vi "Config Panel.vi"(7 "Error In":errorcluster, 10 "MSX-E3711 in":refnum<class "MSX-E3711.lvclass">=refnum) -> (0 "Error Out":errorcluster, 3 "MSX-E3711 out":refnum<class "MSX-E3711.lvclass">)   [LabVIEW 2014, in "MSX-E3711.lvlib" / "MSX-E3711.lvclass"]
doc: "PANEL FRONTAL PARA PRICIPAL DE CONFIGURACION."
uses:
  MSX-E3711Class/MSX-E3711.lvclass
  MSX-E3711Class/MSX-E3711.lvclass/MSX-E3711.ctl
  DriverMasterSync/build/DriverMasterSync.lvlibp/Modules/HAL/DriverMasterSync/DriverMasterSyncClass/DriverMasterSync.lvclass
  API/MSX-E3711_dll.lvlib
panel:
  in  "TempConf":bool
  in  "CountConf":bool
  in  "Activar Temp":bool
  in  "Activar Count":bool
  in  "Activar  Count":bool
  in  "Activar  Temp":bool
  in  "Aplicar":bool
  in  "Cancelar":bool
  in  "Aceptar":bool
  in  "Protection":bool
  in  "Transducer Selection":bool
  in  "Offset":bool
  in  "Gain":bool
  in  "Diagnostic":bool
  in  "Calibration":bool
  in  "Transductores":bool[][](array[boolean])=[[TRUE, FALSE, FALSE, FALSE], [FALSE, FALSE, FALSE, FALSE], [FALSE, FALSE, FALSE, FALSE], [FALSE, FALSE, FALSE, FALSE]]
  in  "Nbr Of Sequence":u64
  in  "Nbr Max Seq To Transfer":u64=800
  in  "Connection Data.IP":string="192.168.2.98"
  # "ADDI-DATA MSX-E3711"
  # "IP Config"
  # "Sequence"
  # "AutoRefresh"
  # "1"
  # "2"
  # "3"
  # "4"
  # "5"
  # "6"
  # "7"
  # "8"
  # "Configuración"
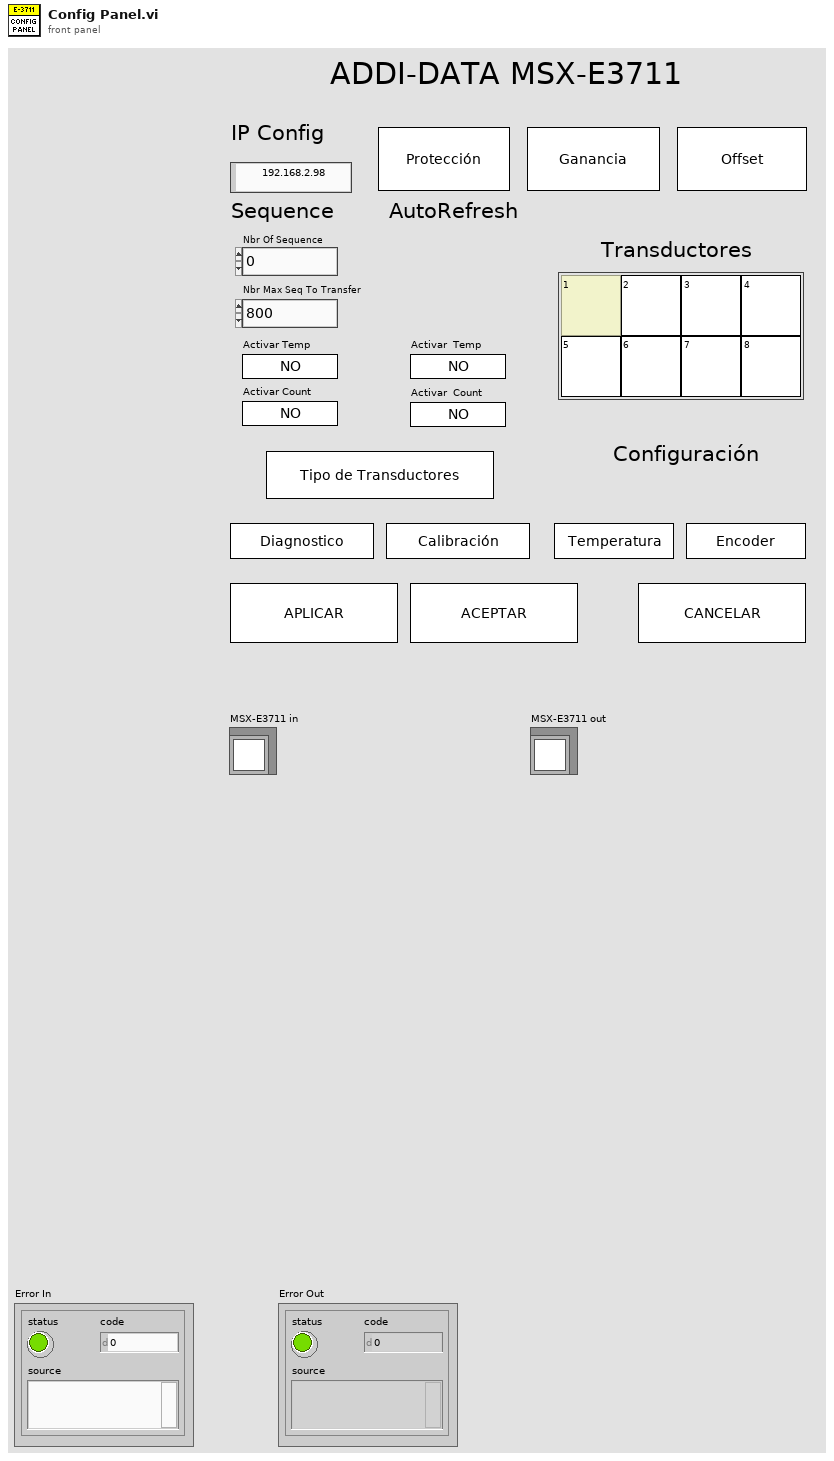
[diagram p1: front panel]
types:
  T1 = typedef "DriverMasterSync.lvlibp/HAL Config Data.ctl" = cluster{"HWSync Index":u32, "Driver Name":string, "Channel Mask":u64}
  T2 = typedef "MSX-E3711_dll.lvlib/Config Data.ctl" = cluster{"Auto Refresh":cluster{"Average Mode":u64, "Average Value":u64, "Trigger Mask":u64, "Trigger Mode":u64, "Hardware Trigger Edge":u64, "Hardware Trigger Count":u64, "By Trigger Nbr Of Seq To Acquire":u64, "Time stamp":bool, "Analog Output(mm)":bool, "Invert value":bool, "Temperature value":bool, "Incremental counter value":bool, "Diff. mode":bool}, "Gain":sgl[], "Offset":sgl[], "Index":u64, "Range":sgl, "Sequence":cluster{"Nbr Of Sequence":u64, "Nbr Max Sequence To Transfer":u64, "Delay Mode":u64, "Delay Time Unit":u64, "Delay Value":u64, "Trigger Mask":u64, "Trigger Mode":u64, "Hardware Trigger Edge":u64, "Hardware Trigger Count":u64, "By Trigger Nbr Of Seq To Acquire":u64, "Time stamp":bool, "Sequence counter information":bool, "Analog Output(mm)":bool, "Invert value":bool, "Temperature value":bool, "Incremental counter value":bool, "Diff. mode":bool}, "Enable DIO":bool, "IncCounter":cluster{"CounterMode":string, "CounterOptionDIRECT  ":bool, "CounterOptionOthers":bool, "CounterClear ":bool, "Cantidad de Pulsos":sgl, "Reducción":sgl}, "IncTemperature":cluster{"ConnectedTempSensor":string, "ConvertMode":string, "InitGainSelection":string, "FrequencySelection":string, "PowerSaveMode":bool, "GainSelection":string, "RefValue":dbl}}
  T3 = cluster{"Average Mode":u64, "Average Value":u64, "Trigger Mask":u64, "Trigger Mode":u64, "Hardware Trigger Edge":u64, "Hardware Trigger Count":u64, "By Trigger Nbr Of Seq To Acquire":u64, "Time stamp":bool, "Analog Output(mm)":bool, "Invert value":bool, "Temperature value":bool, "Incremental counter value":bool, "Diff. mode":bool}
  T4 = cluster{"Nbr Of Sequence":u64, "Nbr Max Sequence To Transfer":u64, "Delay Mode":u64, "Delay Time Unit":u64, "Delay Value":u64, "Trigger Mask":u64, "Trigger Mode":u64, "Hardware Trigger Edge":u64, "Hardware Trigger Count":u64, "By Trigger Nbr Of Seq To Acquire":u64, "Time stamp":bool, "Sequence counter information":bool, "Analog Output(mm)":bool, "Invert value":bool, "Temperature value":bool, "Incremental counter value":bool, "Diff. mode":bool}
  T5 = typedef "MSX-E3711_dll.lvlib/Connection Data.ctl" = cluster{"MX371x refnum":refnum<k24>, "IP":string, "Connection ID ":refnum<k5>, "MXCommon refnum":refnum<k24>}
  T6 = typedef "MSX-E3711_dll.lvlib/Diagnostic Data.ctl" = cluster{"Muestras Diag. Cycle":u32, "Tolerancia Cycle":sgl, "Tolerancia":sgl, "Mask Proteccion T":u64, "Promedio Transd":sgl[]}
  T7 = cluster{"ConnectedTempSensor":string, "ConvertMode":string, "InitGainSelection":string, "FrequencySelection":string, "PowerSaveMode":bool, "GainSelection":string, "RefValue":dbl}
  T8 = cluster{"CounterMode":string, "CounterOptionDIRECT  ":bool, "CounterOptionOthers":bool, "CounterClear ":bool, "Cantidad de Pulsos":sgl, "Reducción":sgl}
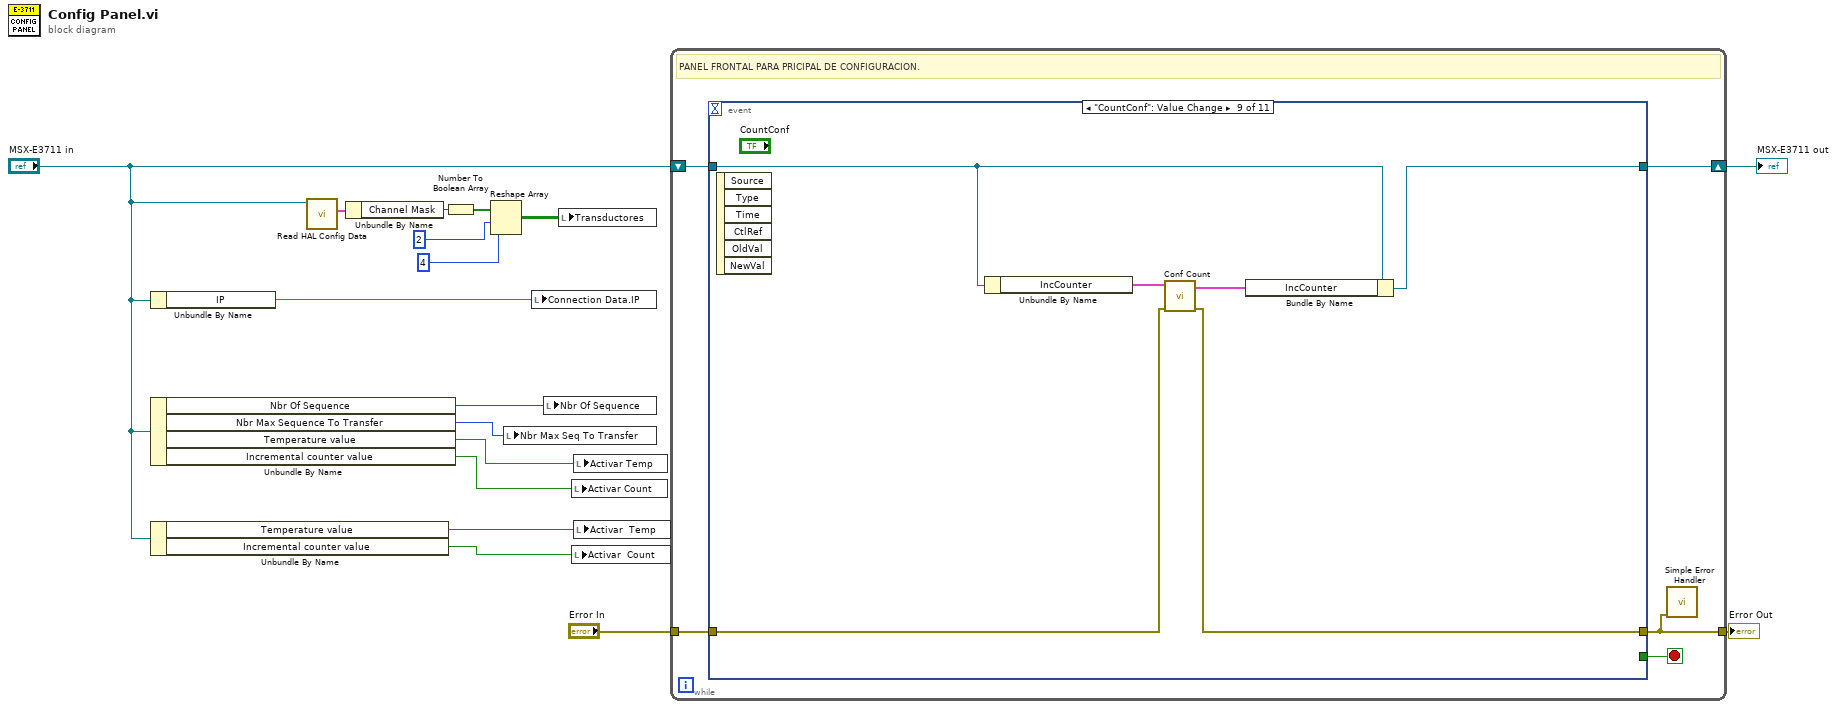
[diagram p0: block diagram]
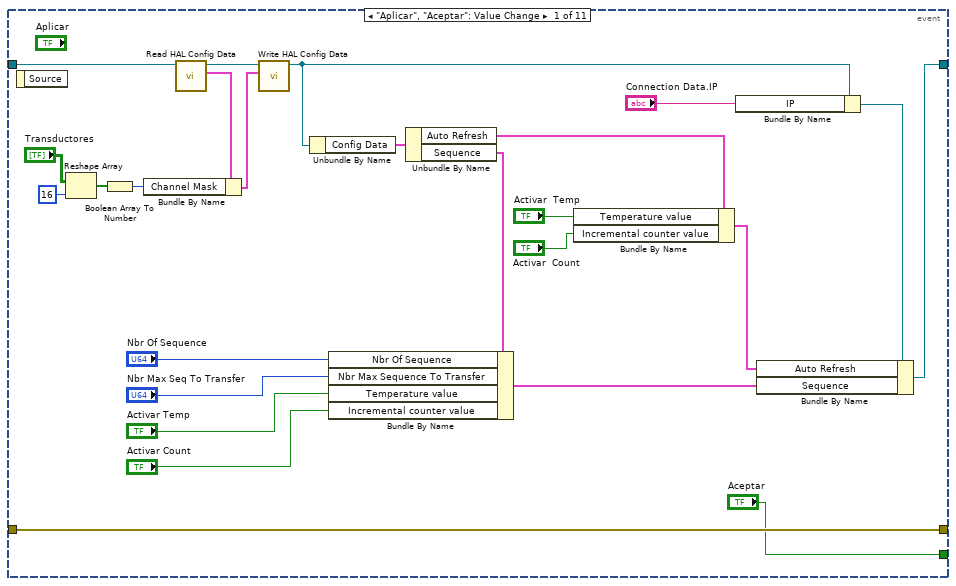
[diagram p2: hidden frame]
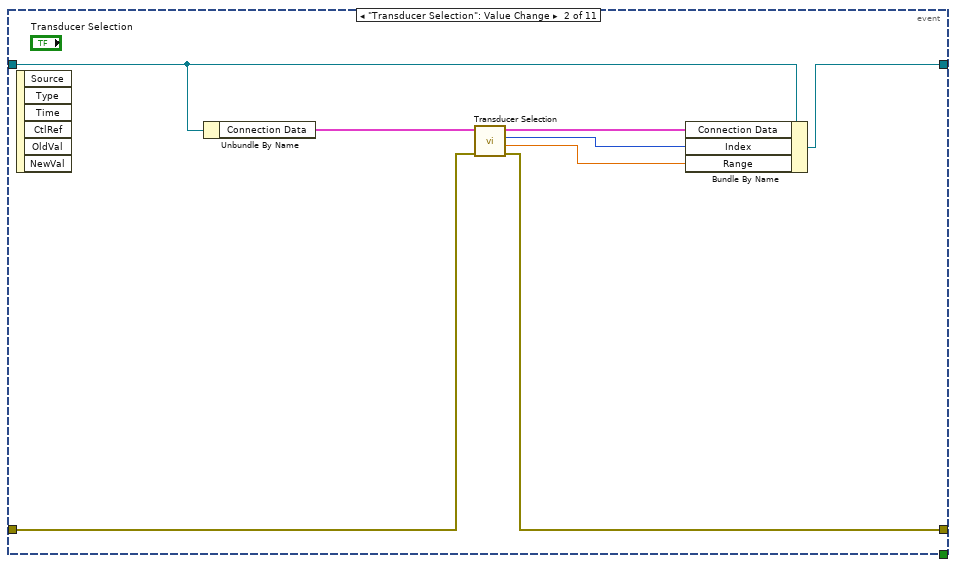
[diagram p3: hidden frame]
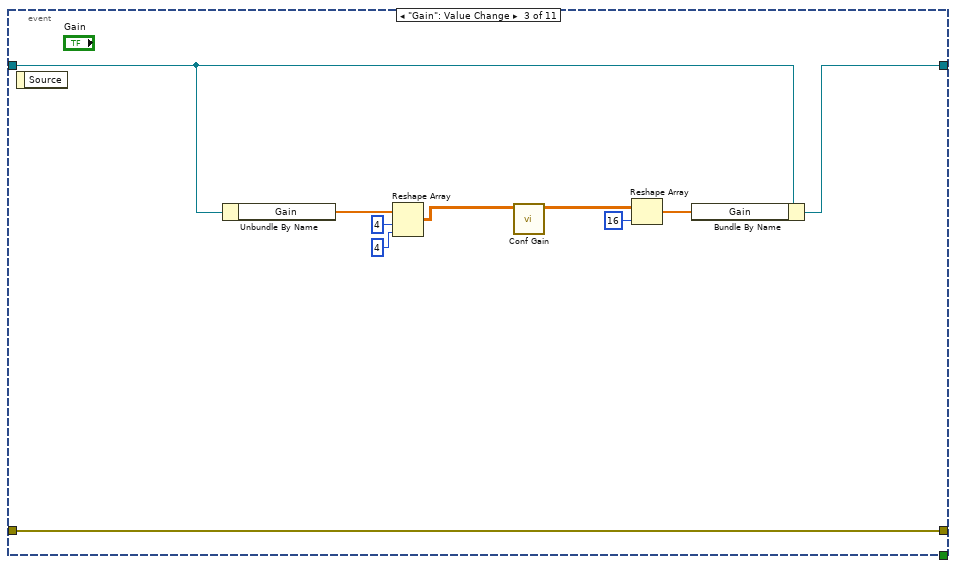
[diagram p4: hidden frame]
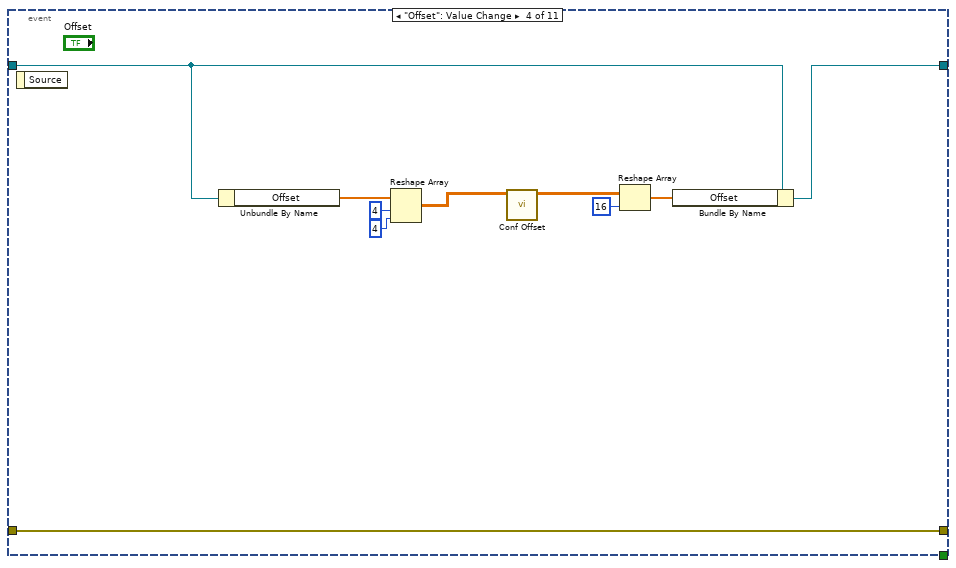
[diagram p5: hidden frame]
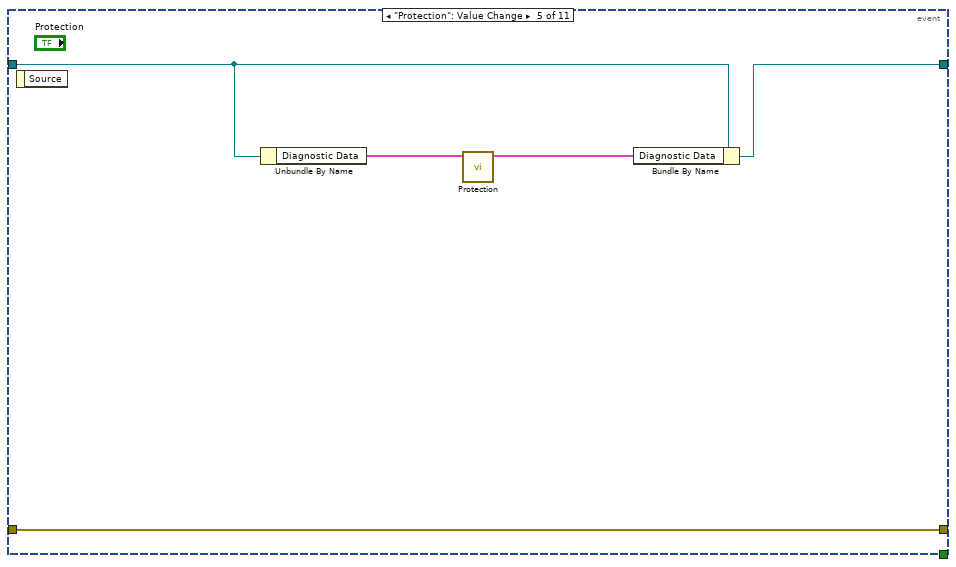
[diagram p6: hidden frame]
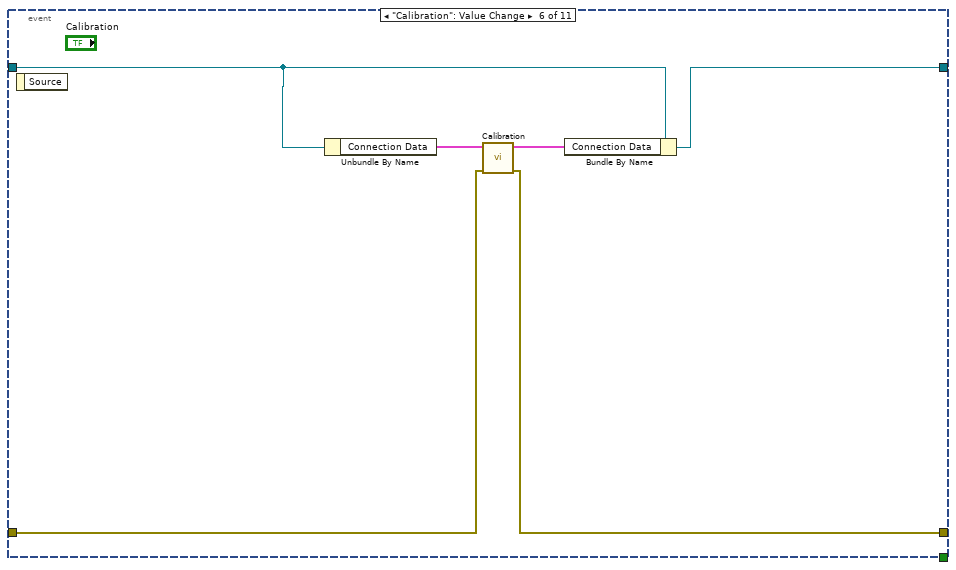
[diagram p7: hidden frame]
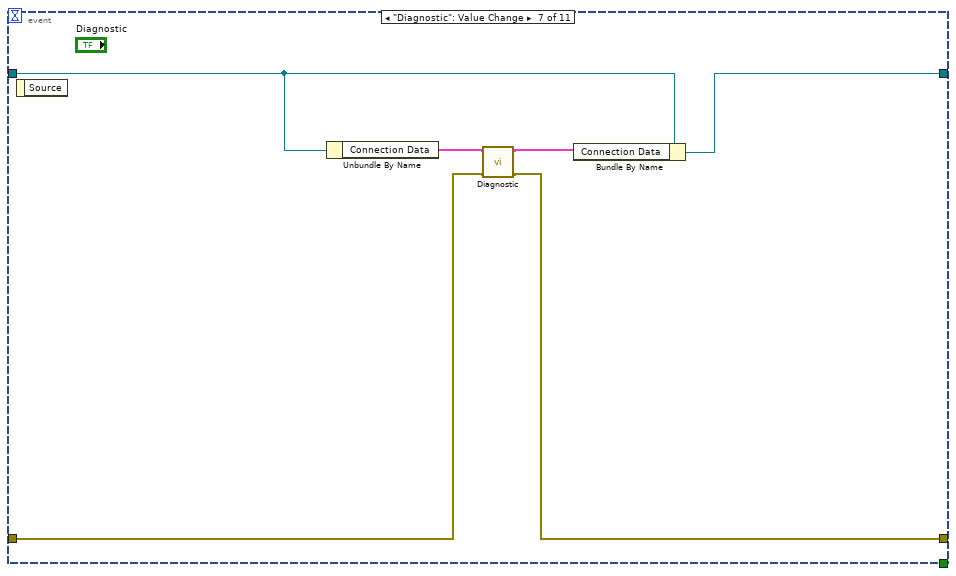
[diagram p8: hidden frame]
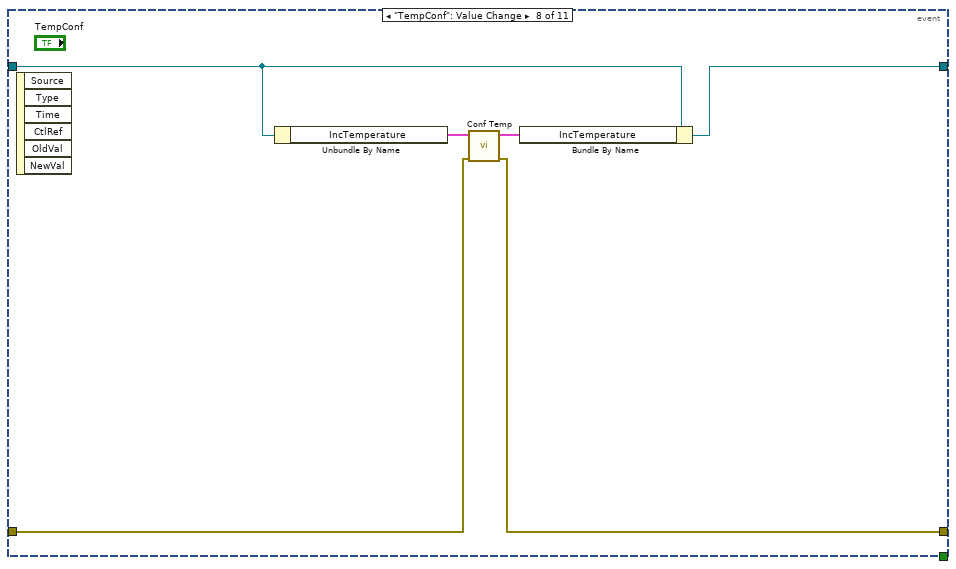
[diagram p9: hidden frame]
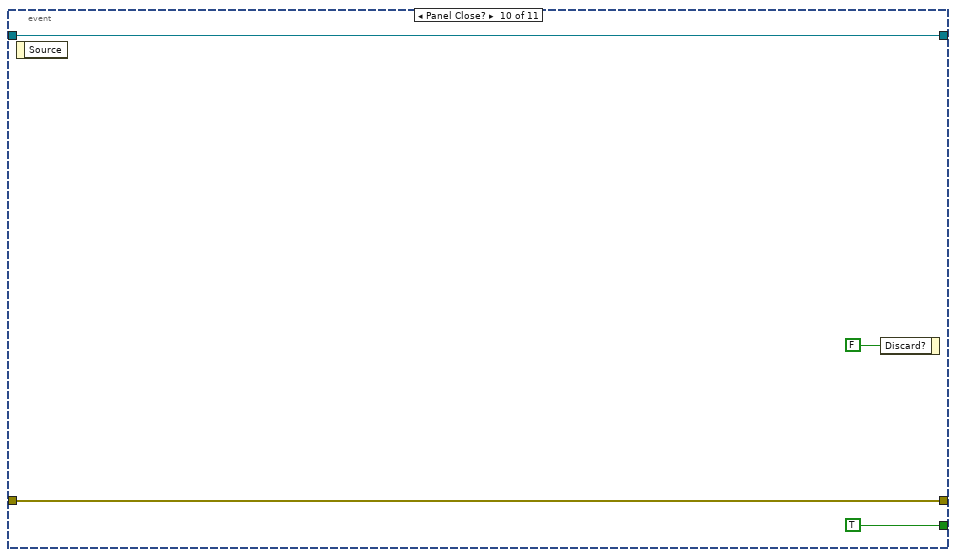
[diagram p10: hidden frame]
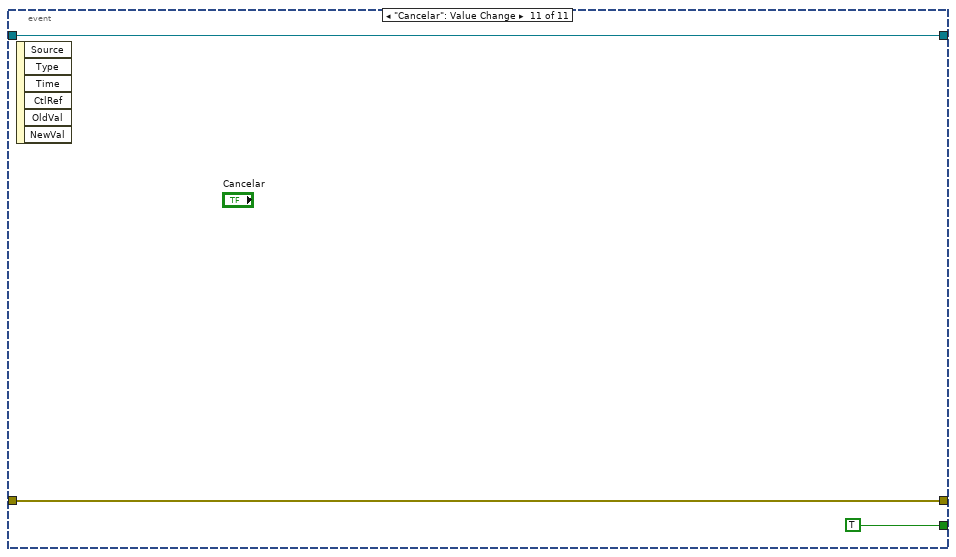
[diagram p11: hidden frame]
diagram:
  n1 = Unbundle By Name("MSX-E3711 in") -> ("IP"=w7:string)
  n2 = Unbundle By Name("MSX-E3711 in") -> ("Nbr Of Sequence"=w9:u64, "Nbr Max Sequence To Transfer"=w8:u64, "Temperature value"=w4:bool, "Incremental counter value"=w3:bool)
  n3 = Unbundle By Name("MSX-E3711 in") -> ("Temperature value"=w2:bool, "Incremental counter value"=w1:bool)
  n4 = call "Read HAL Config Data.vi"("DriverMasterSync in"="MSX-E3711 in") -> ("HAL Config Data"=w15:T1)  [unwired: 8 in, 2 out]
  n5 = Unbundle By Name(w15) -> ("Channel Mask"=w14:u64)
  n6 = Number To Boolean Array(number=w14) -> (Boolean array=w13:bool[])
  n7 = Reshape Array(w13, 2 ("dimension size"), 4 ("dimension size")) -> (w12:bool[][])
  n8 = local write "Nbr Max Seq To Transfer"(w8) -> ()
  n9 = local write "Connection Data.IP"(w7) -> ()
  n10 = local write "Nbr Of Sequence"(w9) -> ()
  n11 = local write "Transductores"(w12) -> ()
  n12 = local write "Activar Count"(w3) -> ()
  n13 = local write "Activar  Count"(w1) -> ()
  n14 = local write "Activar Temp"(w4) -> ()
  n15 = local write "Activar  Temp"(w2) -> ()
  n16 = while {
    tunnel: [w19] -> w17
    tunnel: "Error In" -> [w20]
    shift-right: [w18] -> w6
    shift-left: "MSX-E3711 in" -> [w21]
    stop <- w22 stop-if-true
    # "PANEL FRONTAL PARA PRICIPAL DE CONFIGURACION."
    n17 = event shown="[8] \"CountConf\": Value Change" {
      selector: _ -> [_ _ _ _ _ _ _ _ _ _ _]
      dyn-events: _ -> [_ _ _ _ _ _ _ _ _ _ _]
      timeout: _ -> [_ _ _ _ _ _ _ _ _ _ _]
      tunnel: ["Aceptar" _ _ _ _ _ _ _ _ TRUE ("Cancel Program") TRUE ("Cancel Program")] -> w22
      tunnel: [w45 w54 w63 w73 w78 w86 w91 w96 w99 w108 w111] -> w18
      tunnel: w21 -> [w33 w55 w64 w74 w79 w85 w92 w95 w100 w108 w111]
      tunnel: w20 -> [w39 w52 w65 w75 w80 w81 w87 w94 w103 w107 w110]
      tunnel: [w39 w51 w65 w75 w80 w82 w88 w93 w102 w107 w110] -> w19
      event "Aplicar", "Aceptar": Value Change {
        n18 = event-data() -> ()  [unwired: 1 in, 1 out]
        n19 = Reshape Array("Transductores", 16 ("dimension size")) -> (w38:bool[])
        n20 = Boolean Array To Number(Boolean array=w38) -> (number=w36:u64)
        n21 = call "Read HAL Config Data.vi"("DriverMasterSync in"=w33) -> ("HAL Config Data"=w30:T1, "DriverMasterSync out"=w32:refnum<class "MSX-E3711.lvclass">)  [unwired: 8 in, 1 out]
        n22 = Bundle By Name(cluster=w30, "Channel Mask"=w36) -> (w31:T1)
        n23 = call "Write HAL Config Data.vi"("HAL Config Data"=w31, "DriverMasterSync in"=w32) -> ("DriverMasterSync out"=w29:refnum<class "MSX-E3711.lvclass">)  [unwired: 8 in, 1 out]
        n24 = Unbundle By Name(w29) -> ("Config Data"=w46:T2)
        n25 = Unbundle By Name(w46) -> ("Auto Refresh"=w26:T3, "Sequence"=w41:T4)
        n26 = Bundle By Name(cluster=w41, "Nbr Of Sequence"="Nbr Of Sequence", "Nbr Max Sequence To Transfer"="Nbr Max Seq To Transfer", "Temperature value"="Activar Temp", "Incremental counter value"="Activar Count") -> (w40:T4)
        n27 = Bundle By Name(cluster=w26, "Temperature value"="Activar  Temp", "Incremental counter value"="Activar  Count") -> (w25:T3)
        n28 = Bundle By Name(cluster=w29, "IP"="Connection Data.IP") -> (w44:refnum<class "MSX-E3711.lvclass">)
        n29 = Bundle By Name(cluster=w44, "Auto Refresh"=w25, "Sequence"=w40) -> (w45:refnum<class "MSX-E3711.lvclass">)
      }
      event "Transducer Selection": Value Change {
        n30 = event-data() -> ()  [unwired: 1 in, 6 out]
        n31 = Unbundle By Name(w55) -> ("Connection Data"=w53:T5)
        n32 = call "Transducer Selection.vi"("error in (no error)"=w52, "Connection Data In"=w53) -> ("error out"=w51:errorcluster, "Range"=w48:dbl, "Index"=w49:u64, "Connection Data Out"=w50:T5)  [unwired: 5 in]
        n33 = Bundle By Name(cluster=w55, "Connection Data"=w50, "Index"=w49, "Range"=w48) -> (w54:refnum<class "MSX-E3711.lvclass">)
      }
      event "Gain": Value Change {
        n34 = event-data() -> ()  [unwired: 1 in, 1 out]
        n35 = Unbundle By Name(w64) -> ("Gain"=w62:sgl[])
        n36 = Reshape Array(w62, 4 ("dimension size"), 4 ("dimension size")) -> (w57:sgl[][])
        n37 = call "Conf Gain.vi"("Gain in"=w57) -> ("Gain Out"=w56:sgl[][])  [unwired: 10 in]
        n38 = Reshape Array(w56, 16 ("dimension size")) -> (w58:sgl[])
        n39 = Bundle By Name(cluster=w64, "Gain"=w58) -> (w63:refnum<class "MSX-E3711.lvclass">)
      }
      event "Offset": Value Change {
        n40 = event-data() -> ()  [unwired: 1 in, 1 out]
        n41 = Unbundle By Name(w74) -> ("Offset"=w69:sgl[])
        n42 = Reshape Array(w69, 4 ("dimension size"), 4 ("dimension size")) -> (w67:sgl[][])
        n43 = call "Conf Offset.vi"("Offset in"=w67) -> ("Offset Out"=w66:sgl[][])  [unwired: 10 in]
        n44 = Reshape Array(w66, 16 ("dimension size")) -> (w68:sgl[])
        n45 = Bundle By Name(cluster=w74, "Offset"=w68) -> (w73:refnum<class "MSX-E3711.lvclass">)
      }
      event "Protection": Value Change {
        n46 = event-data() -> ()  [unwired: 1 in, 1 out]
        n47 = Unbundle By Name(w79) -> ("Diagnostic Data"=w77:T6)
        n48 = call "Protection.vi"("Diagnostic Data"=w77) -> ("Diagnostic Data out"=w76:T6)  [unwired: 10 in]
        n49 = Bundle By Name(cluster=w79, "Diagnostic Data"=w76) -> (w78:refnum<class "MSX-E3711.lvclass">)
      }
      event "Calibration": Value Change {
        n50 = event-data() -> ()  [unwired: 1 in, 1 out]
        n51 = Unbundle By Name(w85) -> ("Connection Data"=w84:T5)
        n52 = call "Calibration.vi"("error in (no error)"=w81, "Connection Data In"=w84) -> ("error out"=w82:errorcluster, "Connection Data Out"=w83:T5)  [unwired: 8 in]
        n53 = Bundle By Name(cluster=w85, "Connection Data"=w83) -> (w86:refnum<class "MSX-E3711.lvclass">)
      }
      event "Diagnostic": Value Change {
        n54 = event-data() -> ()  [unwired: 1 in, 1 out]
        n55 = Unbundle By Name(w92) -> ("Connection Data"=w90:T5)
        n56 = call "Diagnostic.vi"("error in (no error)"=w87, "Connection Data In"=w90) -> ("error out"=w88:errorcluster, "Connection Data Out"=w89:T5)  [unwired: 8 in]
        n57 = Bundle By Name(cluster=w92, "Connection Data"=w89) -> (w91:refnum<class "MSX-E3711.lvclass">)
      }
      event "TempConf": Value Change {
        n58 = event-data() -> ()  [unwired: 1 in, 6 out]
        n59 = Unbundle By Name(w95) -> ("IncTemperature"=w98:T7)
        n60 = call "Conf Temp.vi"("error in (no error)"=w94, "IncTemperature"=w98) -> ("error out"=w93:errorcluster, "IncTemperature Out"=w97:T7)  [unwired: 8 in]
        n61 = Bundle By Name(cluster=w95, "IncTemperature"=w97) -> (w96:refnum<class "MSX-E3711.lvclass">)
      }
      event "CountConf": Value Change {
        n62 = event-data() -> ()  [unwired: 1 in, 6 out]
        n63 = Unbundle By Name(w100) -> ("IncCounter"=w104:T8)
        n64 = call "Conf Count.vi"("error in (no error)"=w103, "IncCounter"=w104) -> ("error out"=w102:errorcluster, "IncCounter Out"=w101:T8)  [unwired: 8 in]
        n65 = Bundle By Name(cluster=w100, "IncCounter"=w101) -> (w99:refnum<class "MSX-E3711.lvclass">)
      }
      event Panel Close? {
        n66 = event-data() -> ()  [unwired: 1 in, 1 out]
        n67 = event-data("Discard?"=FALSE) -> ()  [unwired: 1 in, 1 out]
      }
      event "Cancelar": Value Change {
        n68 = event-data() -> ()  [unwired: 1 in, 6 out]
      }
    }
    n69 = call <vilib>:"Simple Error Handler.vi"("error in (no error)"=w19) -> ()  [unwired: 4 in, 5 out]
  }
  "Error Out" <- w17
  "MSX-E3711 out" <- w6
